vi "Add New Reference.vi"(8 "error in (no error)":errorcluster, 10 "Variant":variant, 11 "Data Cluster in":T1) -> (0 "error out":errorcluster, 2 "new reference":i32, 3 "Data Cluster out 2":T1)   [LabVIEW 2025, in "Scripting Server.lvlib"]
uses:
  Scripting Server.lvlib
  Module Data--cluster.ctl
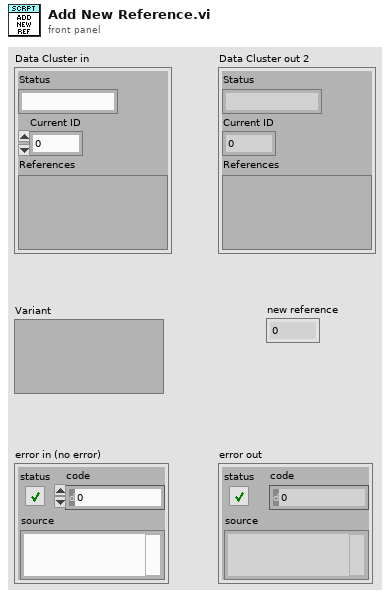
[diagram p1: front panel]
types:
  T1 = typedef "Scripting Server.lvlib/Module Data--cluster.ctl" = cluster{"Status":string, "Current ID":i32, "References":variant}
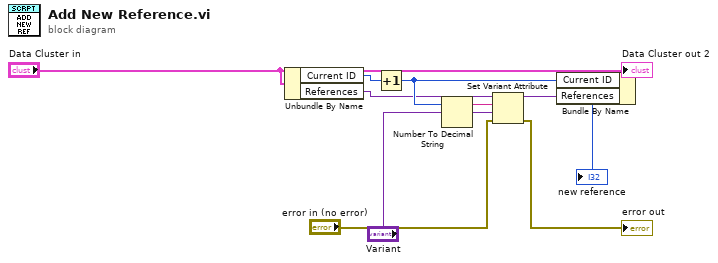
[diagram p0: block diagram]
diagram:
  n1 = Unbundle By Name("Data Cluster in") -> ("Current ID"=w5:i32, "References"=w3:variant)
  n2 = Increment(x=w5) -> (x+1=w6:i32)
  "new reference" <- w6
  n3 = Number To Decimal String(number=w6) -> (decimal integer string=w7:string)  [unwired: 1 in]
  n4 = Set Variant Attribute(Variant=w3, name=w7, value="Variant", error in="error in (no error)") -> (Variant out=w4:variant, error out=→"error out":errorcluster)  [unwired: 1 out]
  n5 = Bundle By Name(cluster="Data Cluster in", "Current ID"=w6, "References"=w4) -> (→"Data Cluster out 2":T1)
